vi "Write_plot-command.vi"(8 "error in (no error)":errorcluster, 10 "plot command":T1, 11 "Plots in":refnum<class "Plots.lvclass">) -> (0 "error out":errorcluster, 3 "Plots out":refnum<class "Plots.lvclass">)   [LabVIEW 2018, in "Plots.lvclass"]
doc: "the VI writes the plot command into the plot command string an into the command queue"
uses:
  Plots.lvclass
  Plots.lvclass/Plots.ctl
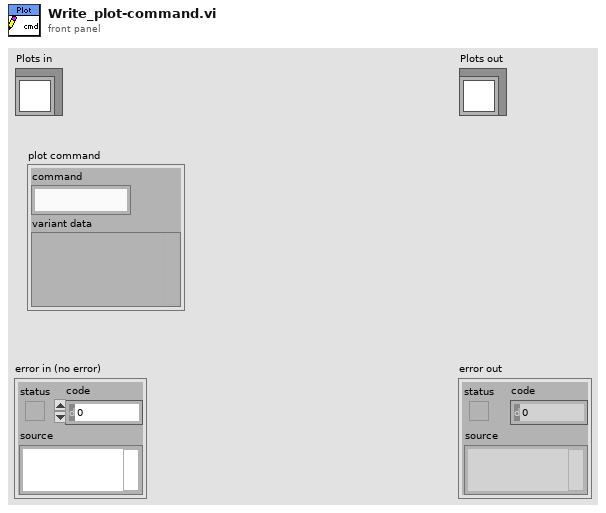
[diagram p1: front panel]
types:
  T1 = cluster{"command":string, "variant data":variant}
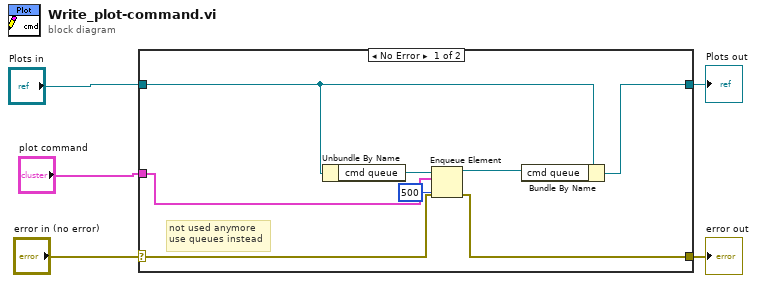
[diagram p0: block diagram]
diagram:
  n1 = case shown="No Error" "error in (no error)" {
    selector: "error in (no error)" -> [w11 w14]
    tunnel: [w10 w14] -> w4
    tunnel: [w8 w15] -> w2
    tunnel: "Plots in" -> [w6 w15]
    tunnel: "plot command" -> [w12 _]
    frame No Error {
      # "not used anymore\nuse queues instead"
      n2 = Unbundle By Name(w6) -> ("cmd queue"=w13:refnum<queue>)
      n3 = Enqueue Element(queue=w13, element=w12, timeout in ms (-1)=500, error in (no error)=w11) -> (queue out=w9:refnum<queue>, error out=w10:errorcluster)  [unwired: 1 out]
      n4 = Bundle By Name(cluster=w6, "cmd queue"=w9) -> (w8:refnum<class "Plots.lvclass">)
    }
    frame Error {
    }
  }
  "error out" <- w4
  "Plots out" <- w2
